vi "main.vi"() -> ()   [LabVIEW 2020]
panel:
  out "PROGRESS":u32(slide) scale=0.0..100.0
  in  "Text Only Button":bool
  in  "Stop":bool
  in  "error in (no error)":errorcluster
  out "error out":errorcluster
  in  "Объекты":T1={"Ускоренно/Реально"=FALSE, "Mashine 1"={"Время на обработку (с)"=40.0, "Процент брака (%)"=4.0}, "Mashine 2"={"Время на обработку (с)"=60.0, "Процент брака (%)"=8.0}, "Кол-во деталей"=500.0, "Robot"={"Время до первого станка"=0.0, "Время до второго станка "=0.0, "Время до урны"=0.0, "Время до коробки"=0.0, "Время между станками"=0.0}}
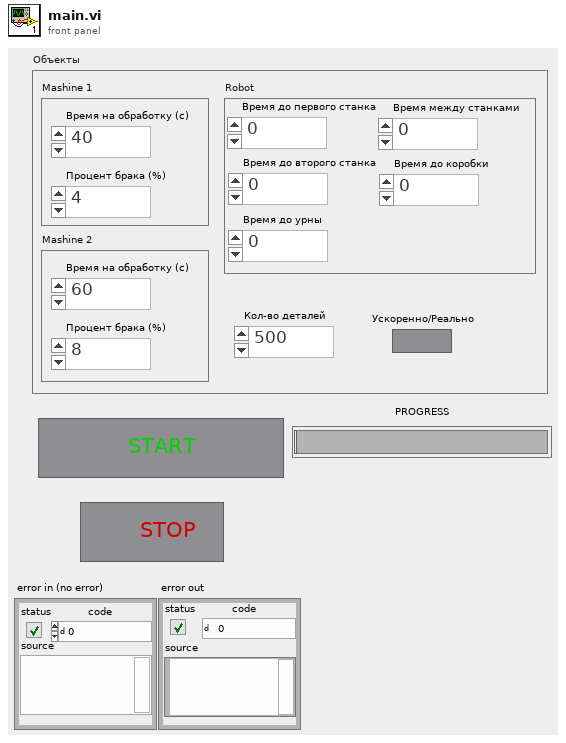
[diagram p1: front panel]
types:
  T1 = cluster{"Ускоренно/Реально":bool, "Mashine 1":cluster{"Время на обработку (с)":dbl, "Процент брака (%)":dbl}, "Mashine 2":cluster{"Время на обработку (с)":dbl, "Процент брака (%)":dbl}, "Кол-во деталей":dbl, "Robot":cluster{"Время до первого станка":dbl, "Время до второго станка ":dbl, "Время до урны":dbl, "Время до коробки":dbl, "Время между станками":dbl}}
  T2 = typedef "Queue elements.ctl" = enum16{"STOP", "START", "BLINK"}
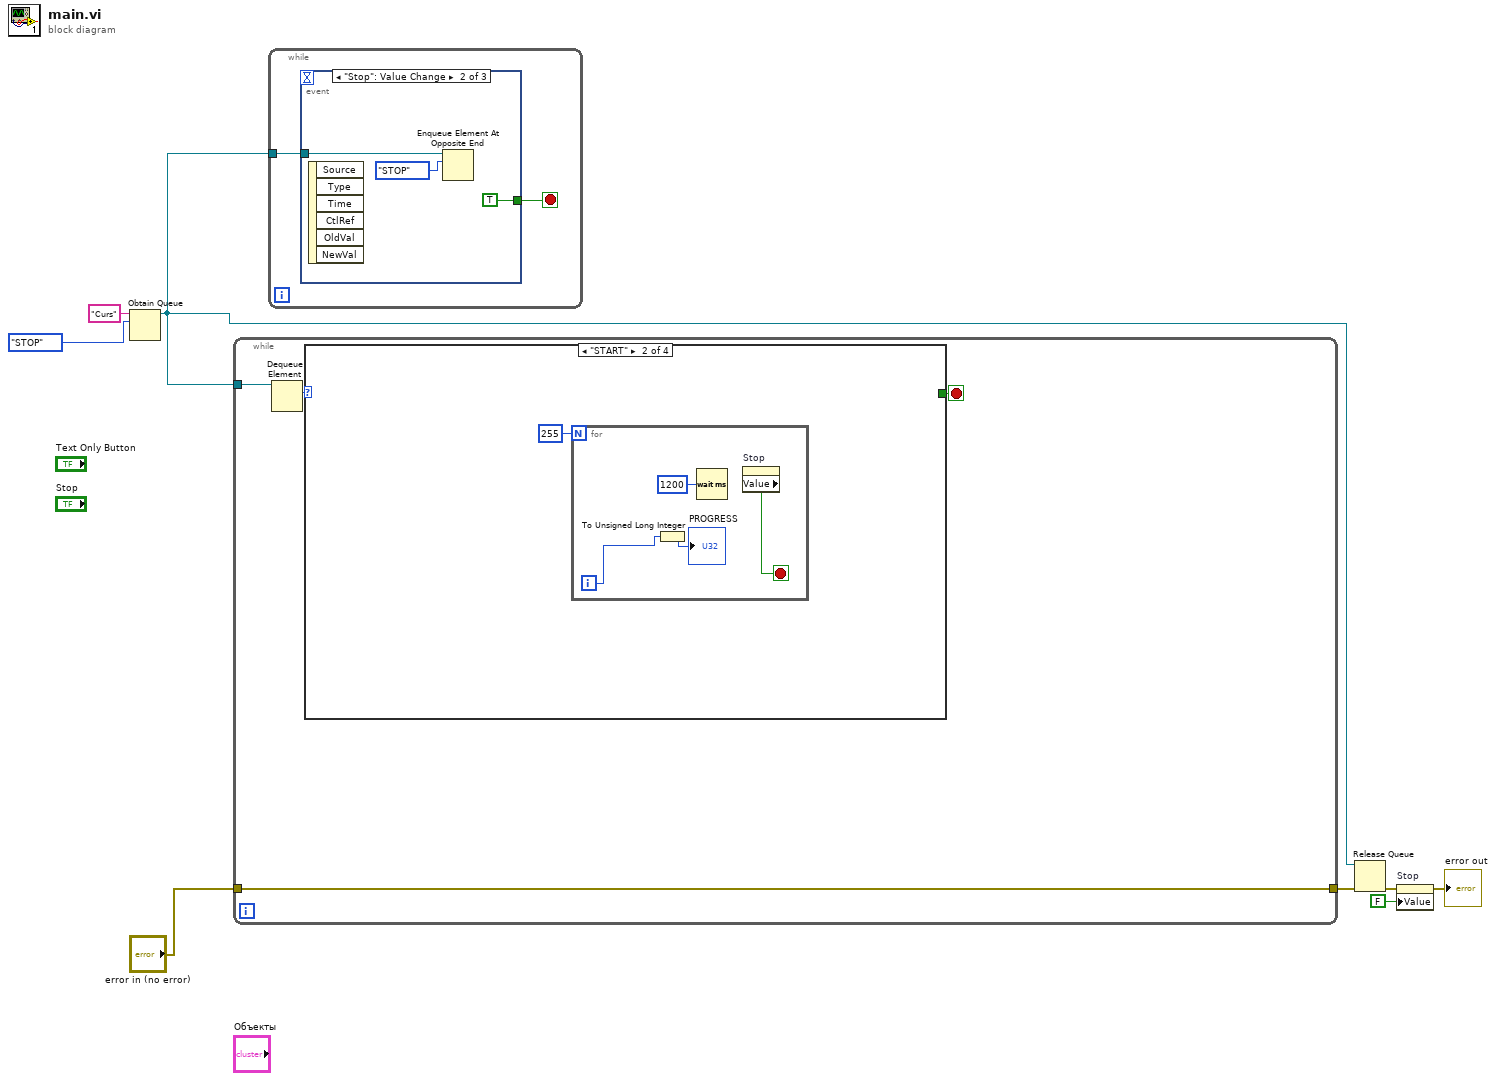
[diagram p0: block diagram]
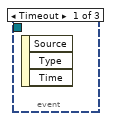
[diagram p2: hidden frame]
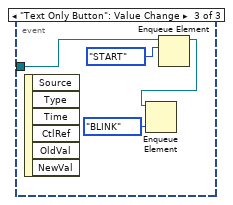
[diagram p3: hidden frame]
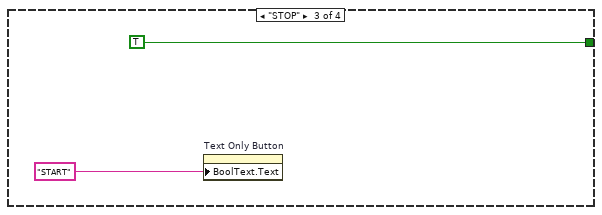
[diagram p5: hidden frame]
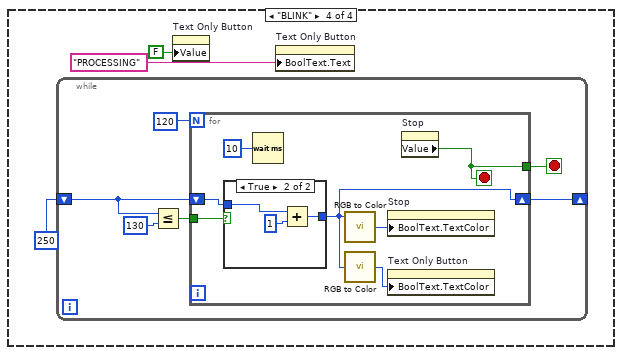
[diagram p6: hidden frame]
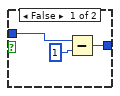
[diagram p7: hidden frame]
diagram:
  n1 = Obtain Queue(name (unnamed)="Curs", element data type=Queue_elements."STOP") -> (queue out=w4:refnum<queue>)  [unwired: 3 in, 2 out]
  n2 = while {
    tunnel: [w12] -> w3
    tunnel: "error in (no error)" -> [w12]
    tunnel: w4 -> [w11]
    stop <- w9 stop-if-true
    n3 = Dequeue Element(queue=w11) -> (element=w10:T2)  [unwired: 2 in, 3 out]
    n4 = case shown="\"START\"" w10 {
      tunnel: [_ _ TRUE _] -> w9
      frame Default {
      }
      frame "START" {
        n5 = for {
          N: 255 -> [_]
          i -> [w16]
          stop <- w15 stop-if-true
          n6 = To Unsigned Long Integer(number=w16) -> (unsigned 32bit integer=→"PROGRESS":u32)
          n7 = Wait (ms)(milliseconds to wait=u32 1200) -> ()  [unwired: 1 out]
          n8 = property on="Stop" class="Bool (strict)"() -> ("Value"=w15:bool)  [unwired: 2 in, 2 out]
        }
      }
      frame "STOP" {
        n9 = property on="Text Only Button" class="Bool (strict)"("BoolText.Text"="START" ("Boolean Text.Text")) -> ()  [unwired: 2 in, 2 out]
      }
      frame "BLINK" {
        n10 = while {
          shift-right: [w26] -> _
          shift-left: u8 250 ("R") -> [w27]
          stop <- w23 stop-if-true
          n11 = Less Or Equal?(x=w27, y=u8 130) -> (x <= y?=w24:bool)
          n12 = for {
            N: 120 -> [_]
            shift-right: [w29] -> w26
            shift-left: w27 -> [w34]
            tunnel: w24 -> [w33]
            tunnel: [w31] -> w23
            stop <- w31 stop-if-true
            n13 = case shown="True" w33 {
              tunnel: [w38 w41] -> w29
              tunnel: w34 -> [w37 w40]
              frame False {
                n14 = Subtract(x=w37, y=u8 1) -> (x-y=w38:u8)
              }
              frame True {
                n15 = Add(x=w40, y=u8 1) -> (x+y=w41:u8)
              }
            }
            n16 = Wait (ms)(milliseconds to wait=u32 10) -> ()  [unwired: 1 out]
            n17 = call <vilib>:"RGB to Color.vi"("R"=w29) -> ("Color"=w35:u32)  [unwired: 2 in]
            n18 = call <vilib>:"RGB to Color.vi"("G"=w29) -> ("Color"=w30:u32)  [unwired: 2 in]
            n19 = property on="Stop" class="Bool (strict)"("BoolText.TextColor"=w35) -> ()  [unwired: 2 in, 2 out]
            n20 = property on="Text Only Button" class="Bool (strict)"("BoolText.TextColor"=w30) -> ()  [unwired: 2 in, 2 out]
            n21 = property on="Stop" class="Bool (strict)"() -> ("Value"=w31:bool)  [unwired: 2 in, 2 out]
          }
        }
        n22 = property on="Text Only Button" class="Bool (strict)"("Value"=FALSE ("Text Only Button")) -> ()  [unwired: 2 in, 2 out]
        n23 = property on="Text Only Button" class="Bool (strict)"("BoolText.Text"="PROCESSING" ("Boolean Text.Text")) -> ()  [unwired: 2 in, 2 out]
      }
    }
  }
  n24 = while {
    tunnel: w4 -> [w43]
    stop <- w42 stop-if-true
    n25 = event shown="[1] \"Stop\": Value Change" {
      selector: _ -> [_ _ _]
      dyn-events: _ -> [_ _ _]
      timeout: _ -> [_ _ _]
      tunnel: w43 -> [_ w45 w49]
      tunnel: [_ TRUE _] -> w42
      event Timeout {
        n26 = event-data() -> ()  [unwired: 1 in, 3 out]
      }
      event "Stop": Value Change {
        n27 = event-data() -> ()  [unwired: 1 in, 6 out]
        n28 = Enqueue Element At Opposite End(queue=w45, element=Queue_elements."STOP") -> ()  [unwired: 2 in, 3 out]
      }
      event "Text Only Button": Value Change {
        n29 = event-data() -> ()  [unwired: 1 in, 6 out]
        n30 = Enqueue Element(queue=w49, element=Queue_elements."START") -> (queue out=w48:refnum<queue>)  [unwired: 2 in, 2 out]
        n31 = Enqueue Element(queue=w48, element=Queue_elements."BLINK") -> ()  [unwired: 2 in, 3 out]
      }
    }
  }
  n32 = Release Queue(queue=w4, error in (no error)=w3) -> (error out=w2:errorcluster)  [unwired: 1 in, 2 out]
  n33 = property on="Stop" class="Bool (strict)"(error in=w2, "Value"=FALSE ("Stop")) -> (error out=→"error out":errorcluster)  [unwired: 1 in, 1 out]
